vi "_script_import_api_doc.vi"(11 "md path":path) -> ()   [LabVIEW 2014]
uses:
  JKI State Machine++.lvlib
panel:
  out "States":string
  out "appended array":path[](array[path])
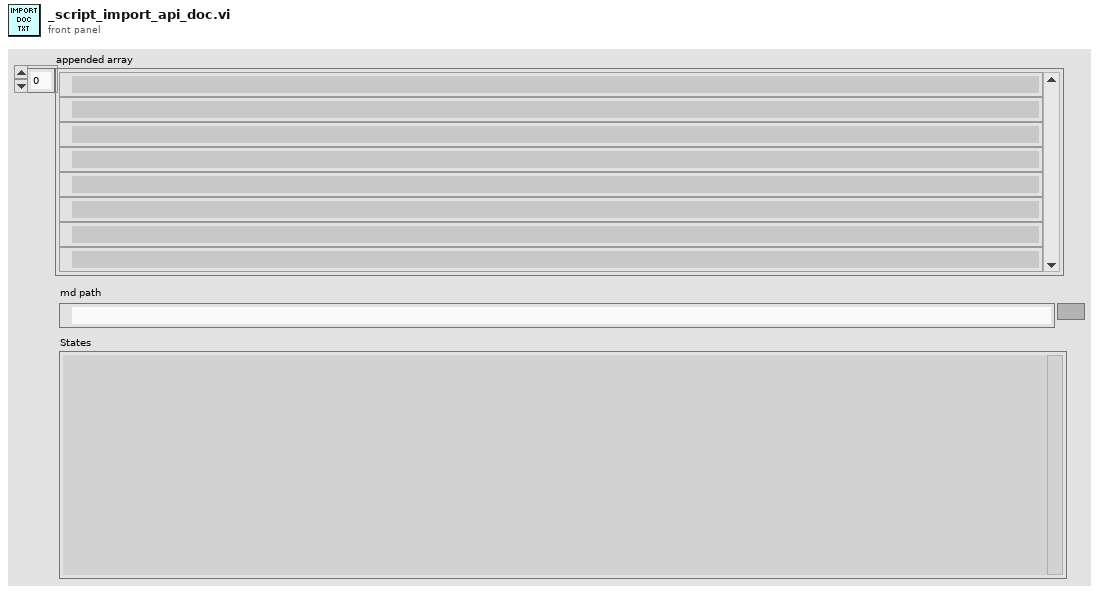
[diagram p1: front panel]
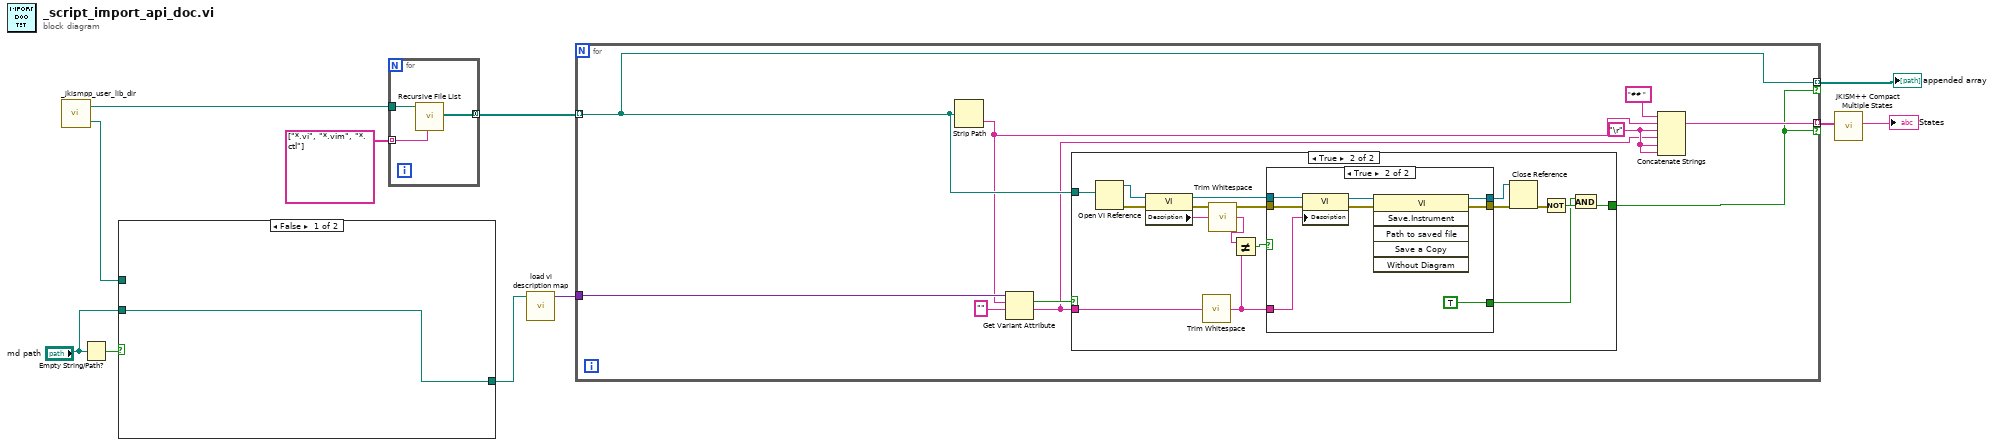
[diagram p0: block diagram]
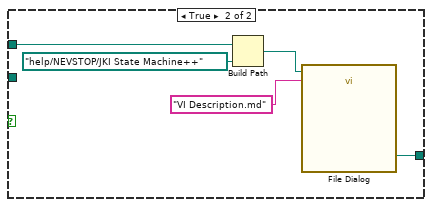
[diagram p2: hidden frame]
diagram:
  n1 = call "_jkismpp_user_lib_dir.vi"() -> ("<LabVIEW>"=w3:path, "jkismpp_user.lib_dir"=w4:path)  [unwired: 2 in]
  n2 = Empty String/Path?(string/path="md path") -> (empty?=w2:bool)
  n3 = case shown="False" w2 {
    tunnel: [w12 w15] -> w7
    tunnel: w3 -> [_ w13]
    tunnel: "md path" -> [w12 _]
    frame False {
    }
    frame True {
      n4 = Build Path(base path=w13, name or relative path=path "help/NEVSTOP/JKI State Machine++" ("Path")) -> (appended path=w16:path)
      n5 = call "File Dialog"("start path"=w16, "default name"="VI Description.md") -> ("selected path"=w15:path)  [unwired: 10 in, 3 out]
    }
  }
  n6 = for {
    tunnel: w4 -> [w20]
    tunnel: string[] ["*.vi", "*.vim", "*.ctl"] -> [w19] mode=indexing
    tunnel: [w18] -> w10 mode=concatenating
    n7 = call <vilib>:"Recursive File List.vi"("pattern"=w19, "Folder Path"=w20) -> ("All Files in Dir"=w18:path[])  [unwired: 5 in, 4 out]
  }
  n8 = call "load vi description map.vi"("Path"=w7) -> ("variant"=w8:variant)  [unwired: 9 in, 1 out]
  n9 = for {
    tunnel: w10 -> [w28] mode=indexing
    tunnel: [w30] -> w9 mode=indexing if=w29
    tunnel: w8 -> [w27]
    tunnel: [w28] -> w5 mode=indexing if=w29
    w25 = "\r"
    n10 = Strip Path(path=w28) -> (name=w22:string)  [unwired: 1 out]
    n11 = Get Variant Attribute(Variant=w27, name=w22, default value (empty Variant)="" ("string")) -> (found=w23:bool, value=w21:string)  [unwired: 1 in, 2 out]
    n12 = case shown="True" w23 {
      tunnel: w28 -> [_ w46]
      tunnel: w21 -> [_ w45]
      tunnel: [_ w32] -> w29
      frame False {
      }
      frame True {
        n13 = Open VI Reference(vi path=w46) -> (vi reference=w39:refnum<vi>, error out=w40:errorcluster)  [unwired: 5 in]
        n14 = property class="VI"(reference=w39, error in=w40) -> (reference out=w37:refnum<vi>, error out=w38:errorcluster, "Description"=w36:string)
        n15 = call <vilib>:"Trim Whitespace.vi"("string"=w45) -> ("trimmed string"=w34:string)  [unwired: 1 in]
        n16 = call <vilib>:"Trim Whitespace.vi"("string"=w36) -> ("trimmed string"=w35:string)  [unwired: 1 in]
        n17 = Not Equal?(x=w35, y=w34) -> (x != y?=w33:bool)
        n18 = case shown="True" w33 {
          tunnel: [w48 w55] -> w44
          tunnel: [w47 w53] -> w43
          tunnel: w34 -> [_ w52]
          tunnel: w38 -> [w48 w51]
          tunnel: w37 -> [w47 w50]
          tunnel: [_ TRUE] -> w31
          frame False {
          }
          frame True {
            n19 = property class="VI"(reference=w50, error in=w51, "Description"=w52) -> (reference out=w54:refnum<vi>, error out=w56:errorcluster)
            n20 = invoke class="VI" method="Save.Instrument"(reference=w54, error in=w56) -> (reference out=w53:refnum<vi>, error out=w55:errorcluster)  [unwired: 4 in, 4 out]
          }
        }
        n21 = Close Reference(reference=w43, error in (no error)=w44) -> (error out=w42:errorcluster)
        n22 = Not(x=w42) -> (.not. x?=w41:bool)
        n23 = And(x=w31, y=w41) -> (x .and. y?=w32:bool)
      }
    }
    n24 = Concatenate Strings("## " ("string"), w22, w25, w21, w25, w25) -> (w30:string)
  }
  "appended array" <- w5
  n25 = call "JKISM++ Compact Multiple States.vi"("States in Lines"=w9) -> ("States"=→"States":string)  [unwired: 9 in]
